vi "Build Excel File.vi"(6 "close report? (T)":bool=TRUE, 7 "Gas":bool, 8 "error in":errorcluster, 9 "Language":T2, 10 "Raw data":string[][](table), 11 "Information":T1) -> (0 "error out":errorcluster, 1 "Excel path":path, 2 "PDF path out":path, 3 "Report path out":path)   [LabVIEW 2016]
uses:
  Controls/Language Control.ctl
  Controls/Information_tab_type.ctl
  <vilib>/Utility/sysdir.llb/System Directory Type.ctl
  <vilib>/Utility/NIReport.llb/NI_report.lvclass
  <vilib>/Utility/NIReport.llb/Excel/NI_Excel.lvclass
  <vilib>/addons/_office/NI_ReportGenerationToolkit.lvlib
panel:
  out "Pass?":bool
  out "rows":i32[](array[numeric])
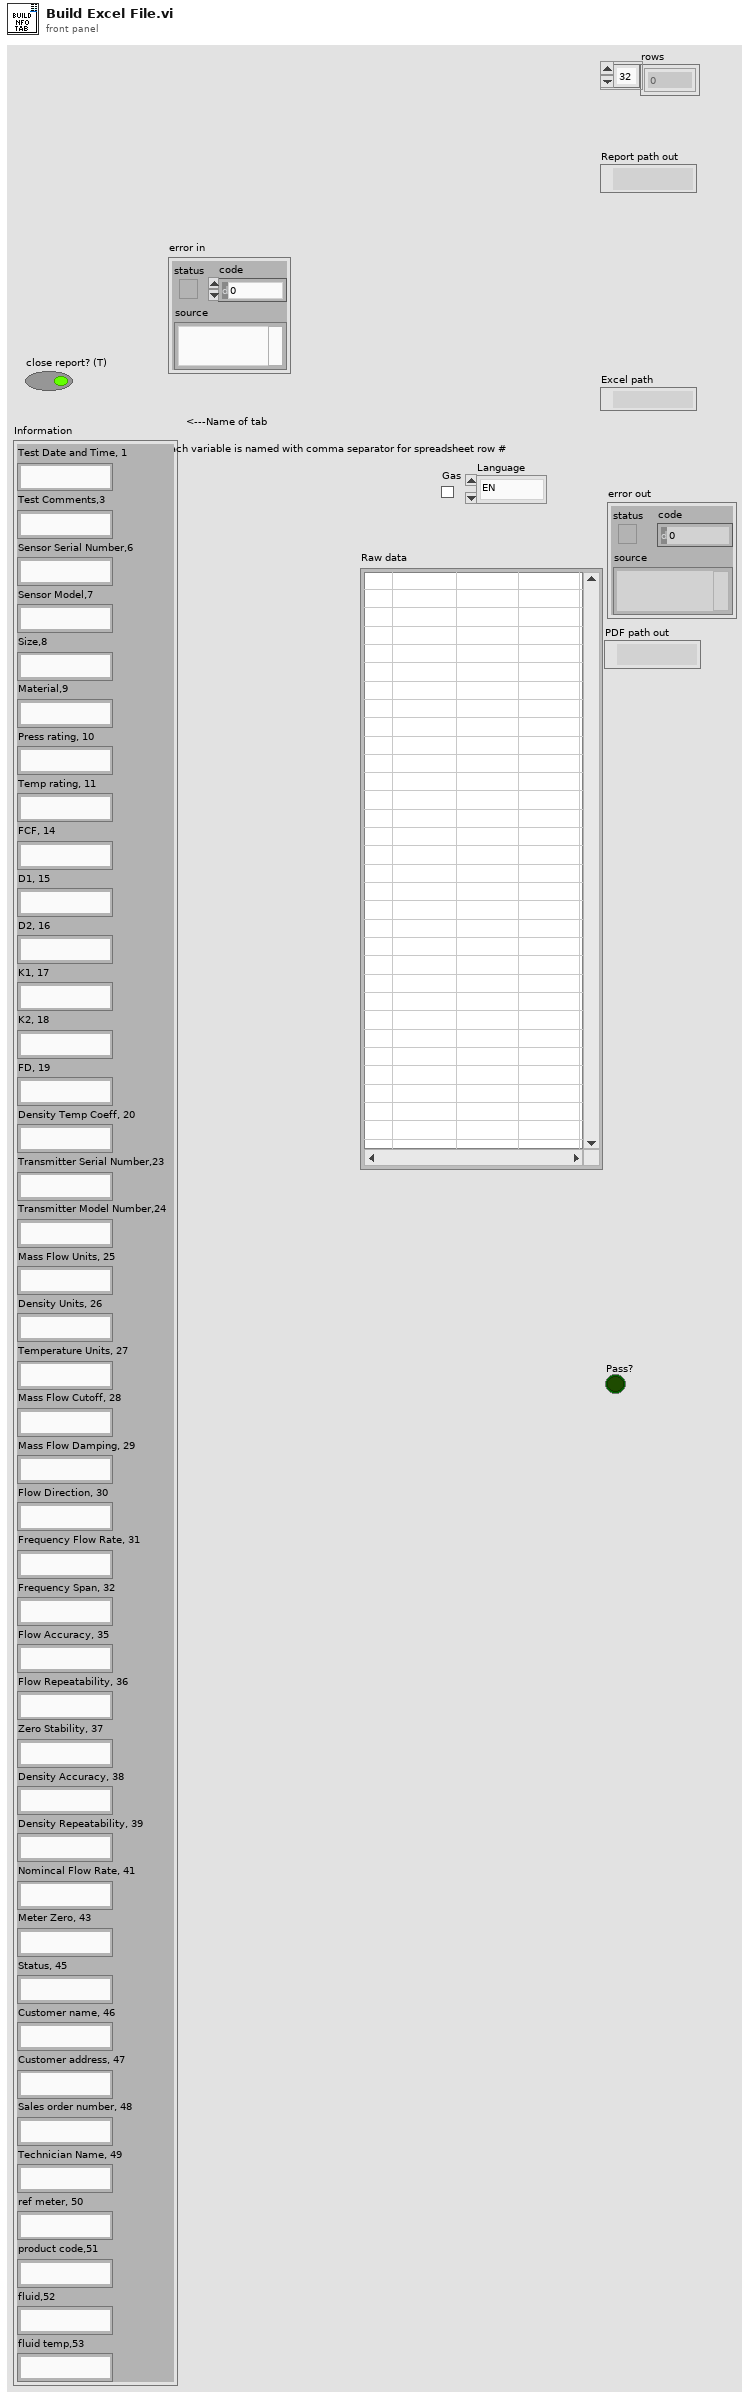
[diagram p1: front panel]
types:
  T1 = typedef "Information_tab_type.ctl" = cluster{"Test Date and Time, 1":string, "Test Comments,3":string, "Sensor Serial Number,6":string, "Sensor Model,7":string, "Size,8":string, "Material,9":string, "Press rating, 10":string, "Temp rating, 11":string, "FCF, 14":string, "D1, 15":string, "D2, 16":string, "K1, 17":string, "K2, 18":string, "FD, 19":string, "Density Temp Coeff, 20":string, "Transmitter Serial Number,23":string, "Transmitter Model Number,24":string, "Mass Flow Units, 25":string, "Density Units, 26":string, "Temperature Units, 27":string, "Mass Flow Cutoff, 28":string, "Mass Flow Damping, 29":string, "Flow Direction, 30":string, "Frequency Flow Rate, 31":string, "Frequency Span, 32":string, "Flow Accuracy, 35":string, "Flow Repeatability, 36":string, "Zero Stability, 37":string, "Density Accuracy, 38":string, "Density Repeatability, 39":string, "Nomincal Flow Rate, 41":string, "Meter Zero, 43":string, "Status, 45":string, "Customer name, 46":string, "Customer address, 47":string, "Sales order number, 48":string, "Technician Name, 49":string, "ref meter, 50":string, "product code,51":string, "fluid,52":string, "fluid temp,53":string}
  T2 = typedef "Language Control.ctl" = enum16{"EN", "ES", "FR", "RU"}
  T3 = typedef "System Directory Type.ctl" = i32
  T4 = enum16{"maximized", "minimized", "normal", "no change"}
  T5 = enum16{"Standard Report", "HTML", "Word", "Excel"}
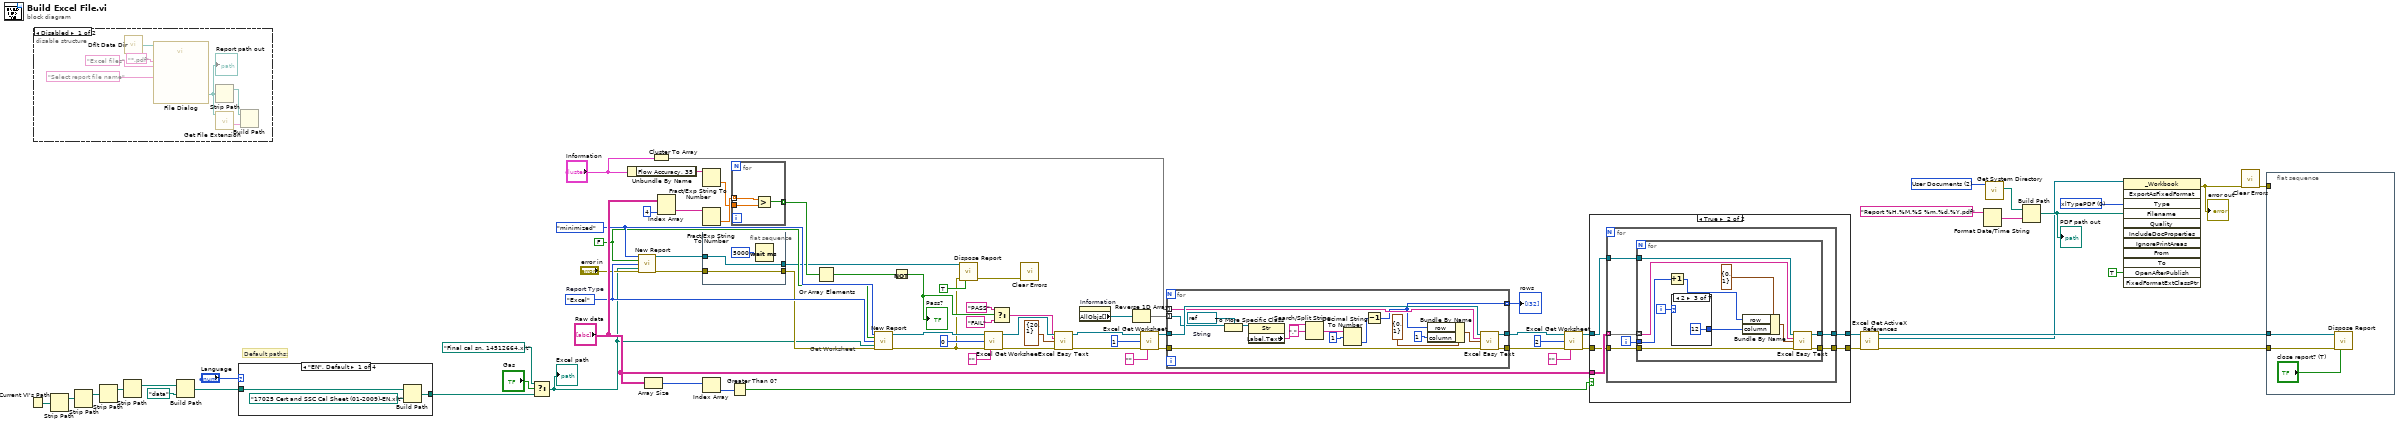
[diagram p0: block diagram]
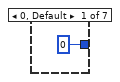
[diagram p3: hidden frame]
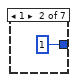
[diagram p4: hidden frame]
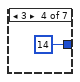
[diagram p5: hidden frame]
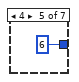
[diagram p6: hidden frame]
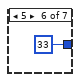
[diagram p7: hidden frame]
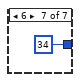
[diagram p8: hidden frame]
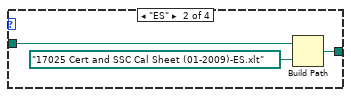
[diagram p10: hidden frame]
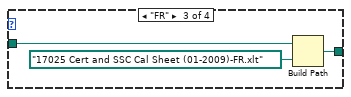
[diagram p11: hidden frame]
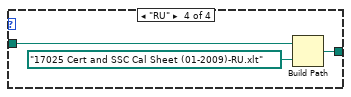
[diagram p12: hidden frame]
diagram:
  w24 = T3 2 items=["User Home"=0, "User Desktop"=1, "User Documents"=2, "User Application Data"=3, "User Preferences"=4, "User Temporary"=5, "Public Documents"=6, "Public Application Data"=7, "Public Preferences"=8, "Public Cache"=13, "System Core Libraries"=9, "System Installed Libraries"=10, "Application Files"=11, "Boot Volume Root"=12] ("system directory type")
  w54 = 0 items=["xlTypePDF", "xlTypeXPS"] ("Type")
  w13 = FALSE ("display alerts? (F)")
  w14 = T4."minimized" ("window state (normal)")
  w12 = T5."Excel"  # Report Type
  # "Default paths:"
  # "Get Worksheet"
  n1 = Current VI's Path() -> (path=w21:path)
  n2 = disable-structure shown="Disabled" {
    frame Disabled {
      n3 = call <vilib>:"Dflt Data Dir.vi"() -> ("App:Default Data Directory"=w82:path)
      n4 = call "File Dialog"("start path"=w82, "prompt"="Select report file name", "pattern (all files)"="*.pdf", "pattern label"="Excel files") -> ("selected path"=w76:path)  [unwired: 8 in, 3 out]
      "Report path out" <- w76
      n5 = Strip Path(path=w76) -> (stripped path=w77:path)  [unwired: 1 out]
      n6 = call <vilib>:"Get File Extension.vi"("file"=w76) -> ("filename without extension"=w78:string)  [unwired: 6 in, 4 out]
      n7 = Build Path(base path=w77, name or relative path=w78) -> ()  [unwired: 1 out]
    }
    frame Enabled {
    }
  }
  n8 = Strip Path(path=w21) -> (stripped path=w20:path)  [unwired: 1 out]
  n9 = Strip Path(path=w20) -> (stripped path=w19:path)  [unwired: 1 out]
  n10 = Strip Path(path=w19) -> (stripped path=w18:path)  [unwired: 1 out]
  n11 = Strip Path(path=w18) -> (stripped path=w17:path)  [unwired: 1 out]
  n12 = Build Path(base path=w17, name or relative path=path "data") -> (appended path=w74:path)
  n13 = case shown="\"EN\", Default" "Language" {
    tunnel: [w85 w88 w91 w94] -> w3
    tunnel: w74 -> [w83 w87 w90 w93]
    frame "EN", Default {
      n14 = Build Path(base path=w83, name or relative path=path "17025 Cert and SSC Cal Sheet (01-2009)-EN.xlt") -> (appended path=w85:path)
    }
    frame "ES" {
      n15 = Build Path(base path=w87, name or relative path=path "17025 Cert and SSC Cal Sheet (01-2009)-ES.xlt") -> (appended path=w88:path)
    }
    frame "FR" {
      n16 = Build Path(base path=w90, name or relative path=path "17025 Cert and SSC Cal Sheet (01-2009)-FR.xlt") -> (appended path=w91:path)
    }
    frame "RU" {
      n17 = Build Path(base path=w93, name or relative path=path "17025 Cert and SSC Cal Sheet (01-2009)-RU.xlt") -> (appended path=w94:path)
    }
  }
  n18 = Select(t=path "Final cal sn. 14512664.xlt", s="Gas", f=w3) -> (s? t:f=w2:path)
  "Excel path" <- w2
  n19 = Unbundle By Name("Information") -> ("Flow Accuracy, 35"=w41:string)
  n20 = call <vilib>:"New Report.vi"("window state (normal)"=w14, "display alerts? (F)"=w13, "report type"=w12, "template (empty)"=w2, "error in (no error)"="error in") -> ("report out"=w9:refnum<class "NI_report.lvclass">, "error out"=w8:errorcluster)  [unwired: 9 in]
  n21 = Array Size(array="Raw data") -> (size(s)=w50:i32[])
  n22 = Cluster To Array(cluster="Information") -> (array=w68:string[])
  n23 = Index Array(array="Raw data", index (col)=4 ("disabled index (col)")) -> (element=w44:string[])  [unwired: 1 in]
  n24 = Fract/Exp String To Number(string=w41) -> (number=w40:dbl)  [unwired: 3 in, 1 out]
  n25 = Fract/Exp String To Number(string=w44) -> (number=w42:dbl[])  [unwired: 3 in, 1 out]
  n26 = flat-sequence {
    tunnel: w9 -> [w97]
    tunnel: w8 -> [w96]
    tunnel: [w97] -> w7
    tunnel: [w96] -> w6
    frame #0 {
      n27 = Wait (ms)(milliseconds to wait=u32 5000) -> ()  [unwired: 1 out]
    }
  }
  n28 = Index Array(array=w50) -> (element=w48:i32)  [unwired: 1 in]
  n29 = Greater Than 0?(x=w48) -> (x > 0?=w49:bool)
  n30 = for {
    tunnel: w42 -> [w100] mode=indexing
    tunnel: w40 -> [w99]
    tunnel: [w98] -> w39 mode=indexing
    n31 = Greater?(x=w100, y=w99) -> (0:w98:bool)
  }
  n32 = Or Array Elements(Boolean array=w39) -> (logical OR=w38:bool)
  n33 = call <vilib>:"New Report.vi"("window state (normal)"=w14, "display alerts? (F)"=w13, "report type"=w12, "template (empty)"=w2, "error in (no error)"=w6) -> ("report out"=w11:refnum<class "NI_report.lvclass">, "error out"=w5:errorcluster)  [unwired: 9 in]
  n34 = Not(x=w38) -> (.not. x?=w37:bool)
  "Pass?" <- w37
  n35 = call-dynamic "Dispose Report.vi"("report in"=w7, "error in (no error)"=w5, "close report? (T)"=TRUE) -> ("error out"=w15:errorcluster)  [unwired: 12 in]
  n36 = call <vilib>:"Excel Get Worksheet.vi"("report in"=w11, "worksheet index (0)"=0, "error in (no error)"=w5, "name (\"\")"="" ("name (\"\")")) -> ("report out"=w32:refnum<class "NI_report.lvclass">, "error out"=w22:errorcluster)  [unwired: 10 in]
  n37 = Select(t="PASS", s=w37, f="FAIL") -> (s? t:f=w29:string)
  n38 = call <vilib>:"Clear Errors.vi"("error in (no error)"=w15) -> ()  [unwired: 5 in, 2 out]
  n39 = call <vilib>:"Excel Easy Text.vi"("report in"=w32, "text"=w29, "start (-1, -1)"=cluster{"row":i32, "column":i32} {"row"=20, "column"=1}, "error in (no error)"=w22) -> ("report out"=w31:refnum<class "NI_report.lvclass">, "error out"=w30:errorcluster)  [unwired: 7 in, 3 out]
  n40 = property on="Information" class="Clust (strict)"() -> ("AllObjs[]"=w67:refnum<vi>[])  [unwired: 2 in, 2 out]
  n41 = Reverse 1D Array(array=w67) -> (reversed array=w66:refnum<vi>[])
  n42 = call <vilib>:"Excel Get Worksheet.vi"("report in"=w31, "worksheet index (0)"=1, "error in (no error)"=w30, "name (\"\")"="" ("name (\"\")")) -> ("report out"=w71:refnum<class "NI_report.lvclass">, "error out"=w72:errorcluster)  [unwired: 10 in]
  n43 = for {
    tunnel: w71 -> [w117]
    tunnel: w72 -> [w116]
    tunnel: [w115] -> w62
    tunnel: [w114] -> w63
    tunnel: w68 -> [w113] mode=indexing
    tunnel: w66 -> [w103] mode=indexing
    tunnel: [w101] -> w47 mode=indexing
    w112 = refnum<vi> refnum  # String
    n44 = To More Specific Class(target class=w112, reference=w103) -> (specific class reference=w111:refnum<vi>)  [unwired: 1 in, 1 out]
    n45 = property class="Str"(reference=w111) -> ("Label.Text"=w110:string)  [unwired: 1 in, 2 out]
    n46 = Search/Split String(string=w110, search string/char (-)=",") -> (match + rest of string=w108:string)  [unwired: 1 in, 2 out]
    n47 = Decimal String To Number(string=w108, offset=1) -> (number=w106:i32)  [unwired: 1 in, 1 out]
    n48 = Decrement(x=w106) -> (x-1=w101:i32)
    n49 = Bundle By Name(cluster=cluster{"row":i32, "column":i32} {"row"=0, "column"=1} ("start (-1, -1)"), "row"=w101, "column"=1) -> (w104:cluster{"row":i32, "column":i32})
    n50 = call <vilib>:"Excel Easy Text.vi"("report in"=w117, "text"=w113, "start (-1, -1)"=w104, "error in (no error)"=w116) -> ("report out"=w114:refnum<class "NI_report.lvclass">, "error out"=w115:errorcluster)  [unwired: 7 in, 3 out]
  }
  "rows" <- w47
  n51 = call <vilib>:"Excel Get Worksheet.vi"("report in"=w63, "worksheet index (0)"=2, "error in (no error)"=w62, "name (\"\")"="" ("name (\"\")")) -> ("report out"=w61:refnum<class "NI_report.lvclass">, "error out"=w60:errorcluster)  [unwired: 10 in]
  n52 = case shown="True" w49 {
    tunnel: "Raw data" -> [_ w124]
    tunnel: w61 -> [w119 w123]
    tunnel: w60 -> [w118 w122]
    tunnel: [w119 w121] -> w59
    tunnel: [w118 w120] -> w51
    frame False {
    }
    frame True {
      n53 = for {
        tunnel: w124 -> [w129] mode=indexing
        tunnel: w123 -> [w128]
        tunnel: [w127] -> w121
        tunnel: w122 -> [w126]
        tunnel: [w125] -> w120
        i -> [w130]
        n54 = for {
          tunnel: w130 -> [w139]
          tunnel: w129 -> [w136] mode=indexing
          tunnel: w128 -> [w134]
          tunnel: [w133] -> w127
          tunnel: w126 -> [w132]
          tunnel: [w131] -> w125
          i -> [w137]
          n55 = Increment(x=w139) -> (x+1=w138:i32)
          n56 = case shown="2" w137 {
            tunnel: [0 ("column") 1 ("column") 12 ("column") 14 ("column") 6 ("column") 33 ("column") 34 ("column")] -> w135
            frame 0, Default {
            }
            frame 1 {
            }
            frame 2 {
            }
            frame 3 {
            }
            frame 4 {
            }
            frame 5 {
            }
            frame 6 {
            }
          }
          n57 = Bundle By Name(cluster=cluster{"row":i32, "column":i32} {"row"=0, "column"=1} ("start (-1, -1)"), "row"=w138, "column"=w135) -> (w140:cluster{"row":i32, "column":i32})
          n58 = call <vilib>:"Excel Easy Text.vi"("report in"=w134, "text"=w136, "start (-1, -1)"=w140, "error in (no error)"=w132) -> ("report out"=w133:refnum<class "NI_report.lvclass">, "error out"=w131:errorcluster)  [unwired: 7 in, 3 out]
        }
      }
    }
  }
  n59 = call <vilib>:"Excel Get ActiveX References.vi"("report in"=w59, "error in (no error)"=w51) -> ("report out"=w58:refnum<class "NI_report.lvclass">, "Excel._Workbook"=w52:refnum<k7>, "error out"=w27:errorcluster)  [unwired: 7 in, 4 out]
  n60 = Format Date/Time String(time format string (%c)="Report %H.%M.%S %m.%d.%Y.pdf") -> (date/time string=w56:string)  [unwired: 2 in]
  n61 = call <vilib>:"Get System Directory.vi"("system directory type"=w24) -> ("system directory"=w23:path)  [unwired: 10 in]
  n62 = Build Path(base path=w23, name or relative path=w56) -> (appended path=w55:path)
  "PDF path out" <- w55
  n63 = invoke class="_Workbook" method="ExportAsFixedFormat"(reference=w52, "Type"=w54, "Filename"=w55, "OpenAfterPublish"=TRUE) -> (error out=w25:errorcluster)  [unwired: 8 in, 11 out]
  "error out" <- w25
  n64 = call <vilib>:"Clear Errors.vi"("error in (no error)"=w25) -> ("error out"=w26:errorcluster)  [unwired: 5 in, 1 out]
  n65 = flat-sequence {
    tunnel: w58 -> [w150]
    tunnel: w27 -> [w149]
    tunnel: w26 -> [_]
    frame #0 {
      n66 = call-dynamic "Dispose Report.vi"("report in"=w150, "error in (no error)"=w149, "close report? (T)"="close report? (T)") -> ()  [unwired: 12 in, 1 out]
    }
  }
